vi "SET_ActiveData.vi"(8 "error in (no error)":errorcluster, 10 "Active Data":variant, 11 "FakedArray.lvclass in":refnum<class "FakedArray.lvclass">) -> (0 "error out":errorcluster, 3 "FakedArray.lvclass out":refnum<class "FakedArray.lvclass">)   [LabVIEW 2020, in "FakedArray.lvclass"]
uses:
  FakedArray.lvclass
  FakedArray.lvclass/FakedArray.ctl
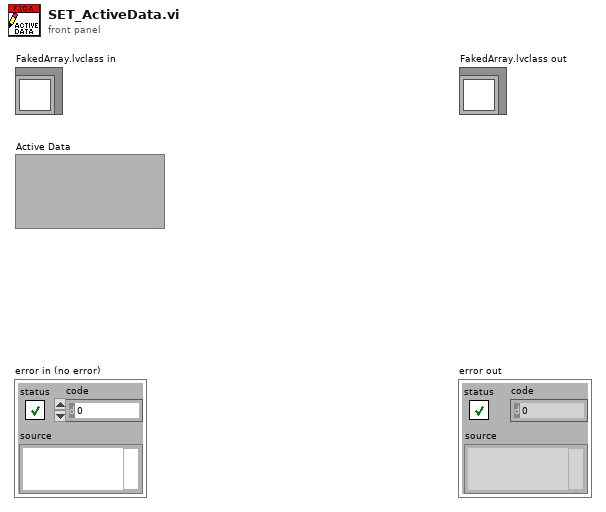
[diagram p1: front panel]
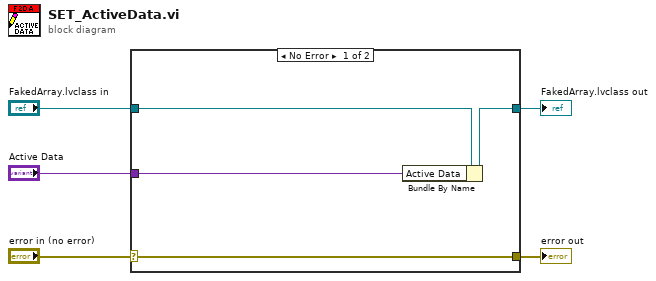
[diagram p0: block diagram]
diagram:
  n1 = case shown="No Error" "error in (no error)" {
    selector: "error in (no error)" -> [w9 w10]
    tunnel: [w9 w10] -> w4
    tunnel: [w7 w11] -> w2
    tunnel: "FakedArray.lvclass in" -> [w8 w11]
    tunnel: "Active Data" -> [w6 _]
    frame No Error {
      n2 = Bundle By Name(cluster=w8, "Active Data"=w6) -> (w7:refnum<class "FakedArray.lvclass">)
    }
    frame Error {
    }
  }
  "error out" <- w4
  "FakedArray.lvclass out" <- w2
